vi "Camera Setup.vi"(8 "error in (no error)":errorcluster, 11 "Camera Input":string="USB 0") -> (0 "error out":errorcluster, 3 "output cluster":T3)   [LabVIEW 2016]
uses:
  <vilib>/Rock Robotics/WPI/Camera/WPI_CameraImageSize.ctl
  <vilib>/vision/Image Controls.llb/IMAQ Image.ctl
  <vilib>/Rock Robotics/WPI/Camera/WPI_CameraDevRef.ctl
  <vilib>/Rock Robotics/WPI/Camera/WPI_CameraWhite Balance Values.ctl
  <vilib>/Rock Robotics/WPI/Camera/WPI_CameraExposure Values.ctl
  <vilib>/Rock Robotics/WPI/Camera/WPI_CameraFrameRate.ctl
  <vilib>/Rock Robotics/Network Tables/NT Read Number.vi
panel:
  in  "Image Size":T4=enum."320x240"
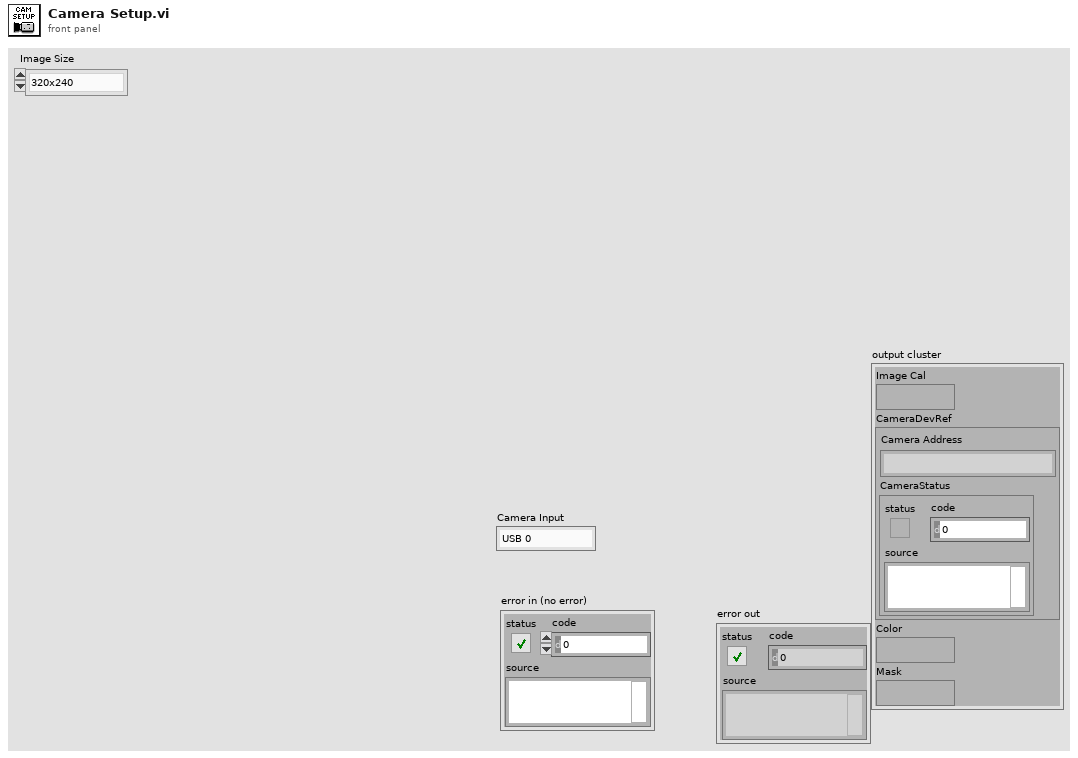
[diagram p1: front panel]
types:
  T1 = typedef "IMAQ Image.ctl" = refnum<image>
  T2 = typedef "WPI_CameraDevRef.ctl" = cluster{"Camera Address":string, "CameraStatus":errorcluster}
  T3 = cluster{"Image Cal":T1, "CameraDevRef":T2, "Color":T1, "Mask":T1}
  T4 = typedef "WPI_CameraImageSize.ctl" = enum16{"640x480", "320x240", "160x120", "Custom"}
  T5 = typedef "WPI_CameraFrameRate.ctl" = u32
  T6 = typedef "WPI_CameraExposure Values.ctl" = enum16{"Auto", "Flicker-free 50 Hz", "Flicker-free 60 Hz", "Hold current", "Custom"}
  T7 = typedef "WPI_CameraWhite Balance Values.ctl" = enum16{"Auto", "Fixed indoor", "Fixed outdoor 1", "Fixed outdoor 2", "Fixed fluorescent 1", "Fixed fluorescent 2", "Hold current", "Custom"}
  T8 = typedef "Image Type" = u32
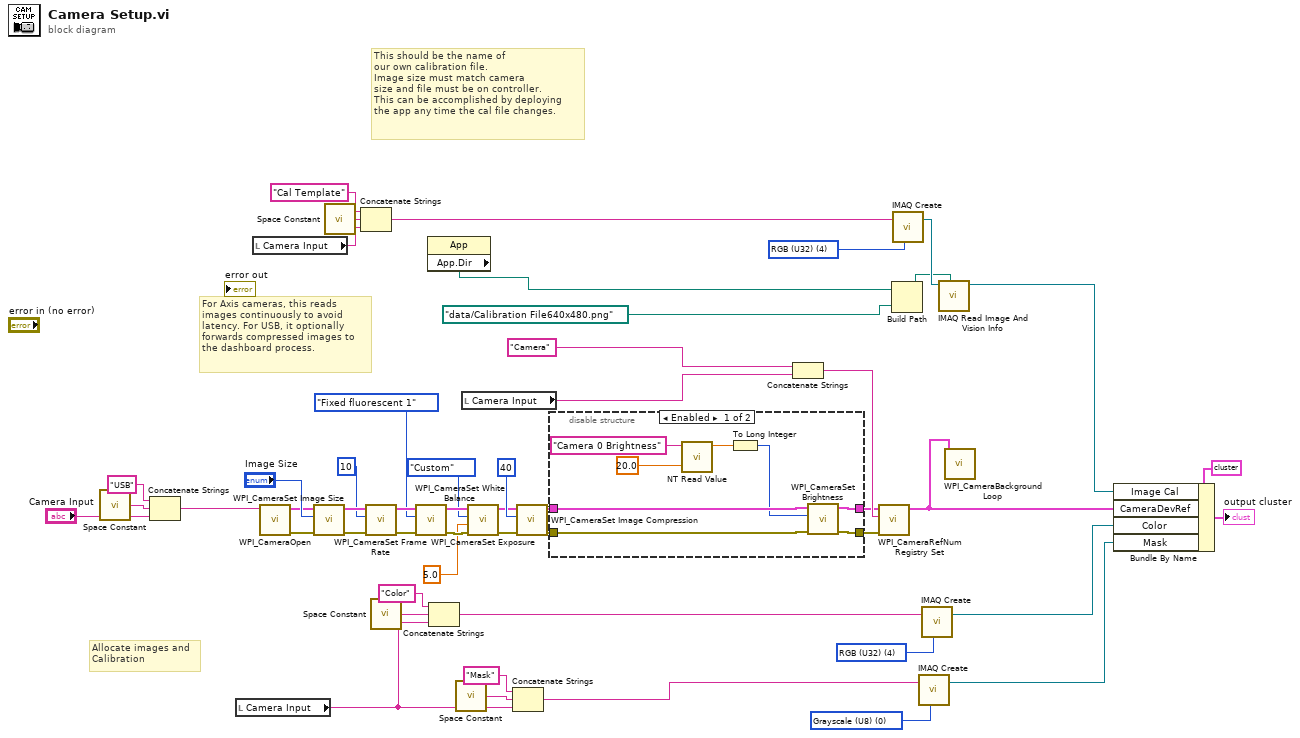
[diagram p0: block diagram]
diagram:
  w49 = T8 4 items=["Grayscale (U8)", "Grayscale (I16)", "Grayscale (SGL)", "Complex (CSG)", "RGB (U32)", "HSL (U32)", "RGB (U64)", "Grayscale (U16)"] ("Image Type")
  w50 = T8 0 items=["Grayscale (U8)", "Grayscale (I16)", "Grayscale (SGL)", "Complex (CSG)", "RGB (U32)", "HSL (U32)", "RGB (U64)", "Grayscale (U16)"] ("Image Type")
  w51 = T8 4 items=["Grayscale (U8)", "Grayscale (I16)", "Grayscale (SGL)", "Complex (CSG)", "RGB (U32)", "HSL (U32)", "RGB (U64)", "Grayscale (U16)"] ("Image Type")
  # "This should be the name of \nour own calibration file.\nImage size must match camera\nsize and file must be on controller.\nThis can be accomplished by deploying\nthe app any time the cal file changes."
  # "For Axis cameras, this reads\nimages continuously to avoid\nlatency. For USB, it optionally\nforwards compressed images to\nthe dashboard process."
  # "Allocate images and\nCalibration"
  n1 = call <vilib>:"Space Constant.vi"() -> ("String"=w26:string)
  n2 = Concatenate Strings("USB", w26, "Camera Input") -> (w27:string)
  n3 = local read "Camera Input"() -> (w18:string)
  n4 = local read "Camera Input"() -> (w15:string)
  n5 = call <vilib>:"WPI_CameraOpen.vi"("Camera Address"=w27) -> ("error out"=w38:errorcluster, "CameraDevRef"=w39:T2)  [unwired: 1 in, 8 out]
  n6 = call <vilib>:"WPI_CameraSet Image Size.vi"("error in (no error)"=w38, "Image Size"="Image Size", "CameraDevRef"=w39) -> ("error out"=w37:errorcluster, "CameraDevRef Out"=w40:T2)  [unwired: 1 in, 6 out]
  n7 = call <vilib>:"Space Constant.vi"() -> ("String"=w17:string)
  n8 = Concatenate Strings("Cal Template" ("Image Name"), w17, w15) -> (w14:string)
  n9 = call <vilib>:"WPI_CameraSet Frame Rate.vi"("error in (no error)"=w37, "Frame Rate (fps)"=T5 10, "CameraDevRef"=w40) -> ("error out"=w36:errorcluster, "CameraDevRef Out"=w42:T2)  [unwired: 7 out]
  n10 = call <vilib>:"Space Constant.vi"() -> ("String"=w24:string)
  n11 = call <vilib>:"WPI_CameraSet White Balance.vi"("error in (no error)"=w36, "White Balance"=WPI_CameraWhite_Balance_Values."Fixed fluorescent 1", "CameraDevRef"=w42) -> ("error out"=w35:errorcluster, "CameraDevRef Out"=w41:T2)  [unwired: 1 in, 6 out]
  n12 = property class="App"() -> ("App.Dir"=w29:path)  [unwired: 2 in, 2 out]
  n13 = Concatenate Strings("Color" ("Image Name"), w24, w18) -> (w19:string)
  n14 = call <vilib>:"Space Constant.vi"() -> ("String"=w21:string)
  n15 = local read "Camera Input"() -> (w12:string)
  n16 = call <vilib>:"WPI_CameraSet Exposure.vi"("error in (no error)"=w35, "Exposure (%)"=5.0, "Exposure"=WPI_CameraExposure_Values."Custom", "CameraDevRef"=w41) -> ("error out"=w34:errorcluster, "CameraDevRef Out"=w43:T2)  [unwired: 6 out]
  n17 = Concatenate Strings("Mask" ("Image Name"), w21, w18) -> (w20:string)
  n18 = call <vilib>:"WPI_CameraSet Image Compression.vi"("error in (no error)"=w34, "Compression"=40, "CameraDevRef"=w43) -> ("error out"=w3:errorcluster, "CameraDevRef Out"=w2:T2)  [unwired: 7 out]
  n19 = disable-structure shown="Enabled" {
    disable-tunnel: [w59 w60] -> w4
    disable-tunnel: w3 -> [w58 w60]
    disable-tunnel: w2 -> [w57 w61]
    disable-tunnel: [w56 w61] -> w1
    frame Enabled {
      n20 = call-poly <vilib>:"NT Read Value.vi"("Default Value"=20.0, "Name"="Camera 0 Brightness") -> ("Numeric"=w54:dbl)  [unwired: 8 in, 1 out]
      n21 = To Long Integer(number=w54) -> (32bit integer=w52:i32)
      n22 = call <vilib>:"WPI_CameraSet Brightness.vi"("error in (no error)"=w58, "Brightness"=w52, "CameraDevRef"=w57) -> ("error out"=w59:errorcluster, "CameraDevRef Out"=w56:T2)  [unwired: 7 out]
    }
    frame Disabled {
    }
  }
  n23 = Concatenate Strings("Camera" ("refnum name"), w12) -> (w11:string)
  n24 = call <vilib>:"WPI_CameraRefNum Registry Set.vi"("error in (no error)"=w4, "refnum name"=w11, "CameraDevRef"=w1) -> ("CameraDevRef"=w9:T2)  [unwired: 1 in, 7 out]
  n25 = Build Path(base path=w29, name or relative path=path "data/Calibration File640x480.png" ("Folder Location")) -> (appended path=w47:path)
  n26 = call "IMAQ Create"("Image Name"=w14, "Image Type"=w49) -> ("New Image"=w48:T1)  [unwired: 2 in, 2 out]
  n27 = call "IMAQ Create"("Image Name"=w20, "Image Type"=w50) -> ("New Image"=w7:T1)  [unwired: 2 in, 2 out]
  n28 = call "IMAQ Create"("Image Name"=w19, "Image Type"=w51) -> ("New Image"=w8:T1)  [unwired: 2 in, 2 out]
  n29 = call "IMAQ Read Image And Vision Info"("File Path"=w47, "Image"=w48) -> ("Image Out"=w10:T1)  [unwired: 7 in, 2 out]
  n30 = call <vilib>:"WPI_CameraBackground Loop.vi"("CameraDevRef"=w9) -> ()  [unwired: 11 in]
  n31 = Bundle By Name(cluster=T3 {"Image Cal"=refnum, "CameraDevRef"={"Camera Address"="", "CameraStatus"={"status"=FALSE, "code"=0, "source"=""}}, "Color"=refnum, "Mask"=refnum}, "Image Cal"=w10, "CameraDevRef"=w9, "Color"=w8, "Mask"=w7) -> (→"output cluster":T3)
